vi "picoharp_generate_lags.vi"(9 "coarseness":i64, 10 "time_end":T1=1 items=["1 ps"=1, "10 ps"=10, "100 ps"=100, "1 ns"=1000, "10 ns"=10000, "100 ns"=100000, "1 us"=1000000, "10 us"=10000000, "100 us"=100000000, "1 ms"=1000000000, "10 ms"=10000000000, "100 ms"=100000000000, "1 s"=1000000000000, "10 s"=10000000000000, "100 s"=100000000000000], 11 "time_start":T1=1 items=["1 ps"=1, "10 ps"=10, "100 ps"=100, "1 ns"=1000, "10 ns"=10000, "100 ns"=100000, "1 us"=1000000, "10 us"=10000000, "100 us"=100000000, "1 ms"=1000000000, "10 ms"=10000000000, "100 ms"=100000000000, "1 s"=1000000000000, "10 s"=10000000000000, "100 s"=100000000000000]) -> (1 "lags":dbl[](array[numeric]), 2 "divisor":dbl[](array[numeric]), 3 "log_bin_edges":dbl[](array[numeric]))   [LabVIEW 2015, in "picoharp.lvclass"]
uses:
  picoharp.lvclass
  Hydraharp/hydraharp/hydraharp_time_decades.ctl
panel:
  out "size(s)":i32
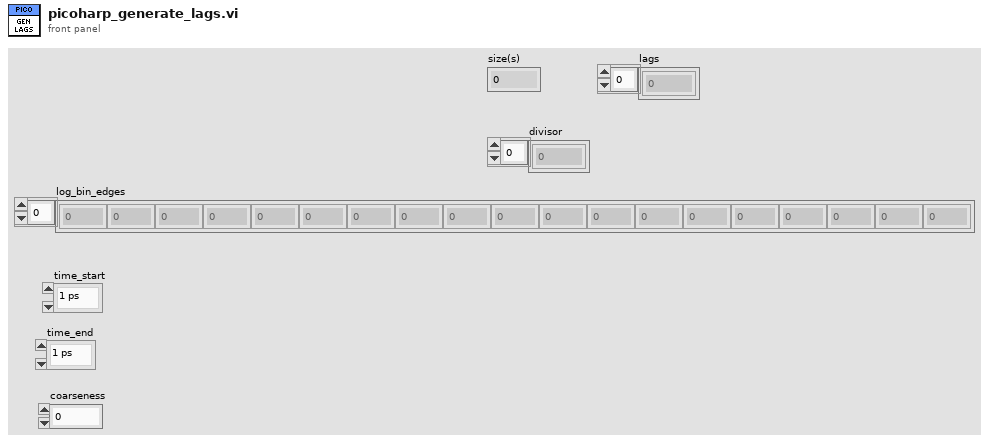
[diagram p1: front panel]
types:
  T1 = typedef "hydraharp_time_decades.ctl" = i64
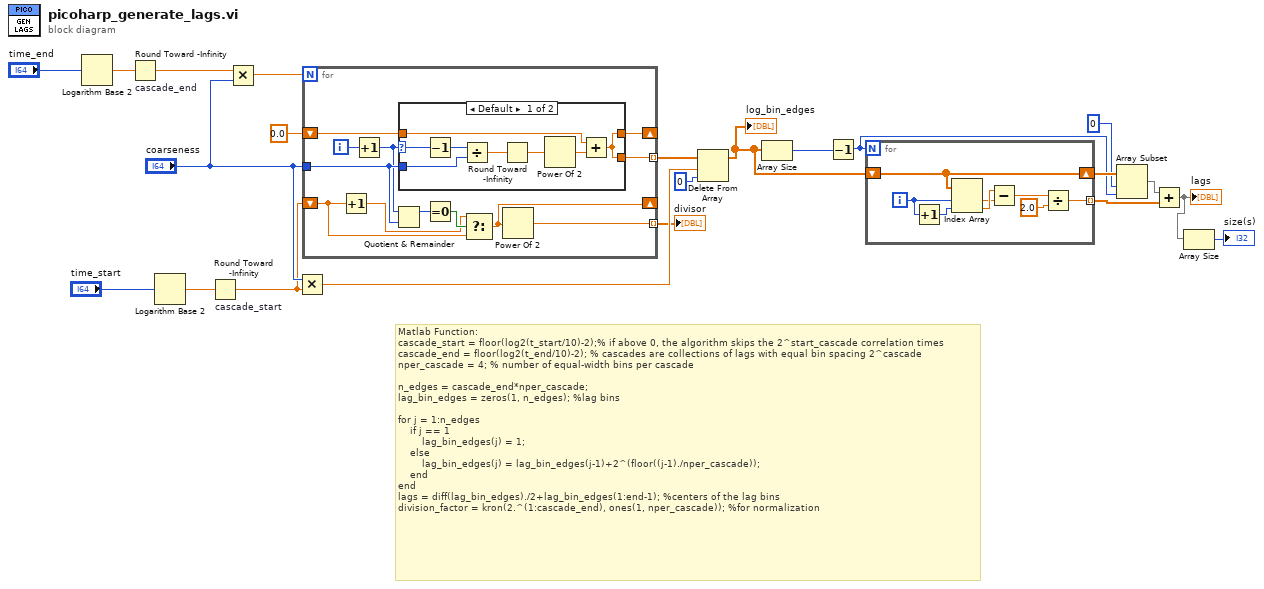
[diagram p0: block diagram]
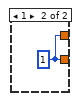
[diagram p2: hidden frame]
diagram:
  # "Matlab Function: \ncascade_start = floor(log2(t_start/10)-2);% if above 0, the algorithm skips the 2^start_cascade correlation times\ncascade_end = floor(log2(t_end/10)-2); % cascades are collections of lags with equal bin spacing 2^cascade\nnper_cascade = 4; % number of equal-width bins per cascade\n\nn_edges = cascade_end*nper_cascade;\nlag_bin_edges = zeros(1, n_edges); %lag bins\n\nfor j = 1:n_edges\n    if j == 1\n        lag_bin_edges(j) = 1;\n    else\n        lag_bin_edges(j) = lag_bin_edges(j-1)+2^(floor((j-1)./nper_cascade));\n    end\nend\nlags = diff(lag_bin_edges)./2+lag_bin_edges(1:end-1); %centers of the lag bins\ndivision_factor = kron(2.^(1:cascade_end), ones(1, nper_cascade)); %for normalization"
  n1 = Logarithm Base 2(1:"time_end") -> (0:w16:dbl)
  n2 = Round Toward -Infinity "cascade_end"(1:w16) -> (0:w22:dbl)
  n3 = Logarithm Base 2(1:"time_start") -> (0:w17:dbl)
  n4 = Round Toward -Infinity "cascade_start"(1:w17) -> (0:w11:dbl)
  n5 = Multiply(x=w22, y="coarseness") -> (x*y=w21:dbl)
  n6 = Multiply(x="coarseness", y=w11) -> (x*y=w13:dbl)
  n7 = for {
    N: w21 -> [_]
    shift-right: [w33] -> _
    shift-left: 0.0 -> [w31]
    tunnel: [w32] -> w14 mode=indexing
    tunnel: "coarseness" -> [w30]
    shift-right: [w24] -> _
    shift-left: w11 -> [w25]
    tunnel: [w23] -> w10 mode=indexing
    i -> [w34]
    n8 = Increment(x=w25) -> (x+1=w26:dbl)
    n9 = Increment(x=w34) -> (x+1=w29:i32)
    n10 = Quotient & Remainder(x=w29, y=w30) -> (x-y*floor(x/y)=w28:i64)  [unwired: 1 out]
    n11 = case shown="Default" w29 {
      selector: w29 -> [w42 _]
      tunnel: [w37 w43] -> w33
      tunnel: [w37 w43] -> w32
      tunnel: w31 -> [w39 _]
      tunnel: w30 -> [w40 _]
      frame Default {
        n12 = Decrement(x=w42) -> (x-1=w41:i32)
        n13 = Divide(x=w41, y=w40) -> (x/y=w36:dbl)
        n14 = Round Toward -Infinity(1:w36) -> (0:w35:dbl)
        n15 = Power Of 2(x=w35) -> (2^x=w38:dbl)
        n16 = Add(x=w39, y=w38) -> (x+y=w37:dbl)
      }
      frame 1 {
        w43 = 1
      }
    }
    n17 = Equal To 0?(x=w28) -> (x = 0?=w27:bool)
    n18 = Select(t=w26, s=w27, f=w25) -> (s? t:f=w24:dbl)
    n19 = Power Of 2(x=w24) -> (2^x=w23:dbl)
  }
  "divisor" <- w10
  n20 = Delete From Array(array=w14, length=w13, index=0) -> (array with subset deleted=w1:dbl[])  [unwired: 1 out]
  "log_bin_edges" <- w1
  n21 = Array Size(array=w1) -> (size(s)=w9:i32)
  n22 = Decrement(x=w9) -> (x-1=w6:i32)
  n23 = for {
    N: w6 -> [_]
    shift-right: [w46] -> w8
    shift-left: w1 -> [w46]
    tunnel: [w47] -> w4 mode=indexing
    i -> [w51]
    n24 = Increment(x=w51) -> (x+1=w50:i32)
    n25 = Index Array(array=w46, index #1=w51, index #2=w50) -> (element #1=w44:dbl, element #2=w45:dbl)
    n26 = Subtract(x=w45, y=w44) -> (x-y=w49:dbl)
    n27 = Divide(x=w49, y=2.0 ("x")) -> (x/y=w47:dbl)
  }
  n28 = Array Subset(array=w8, index=0, length=w6) -> (w5:dbl[])
  n29 = Add(x=w5, y=w4) -> (x+y=w3:dbl[])
  "lags" <- w3
  n30 = Array Size(array=w3) -> (size(s)=→"size(s)":i32)
